vi "Manip_6.vi"() -> ()   [LabVIEW 2020]
uses:
  <vilib>/express/express analysis/Spectral/Block/exnSpectralBlock spectral measurements power poly.vi
  <vilib>/express/express analysis/Spectral/Block/exnSpectralBlock spectral measurements power DDT.vi
  <vilib>/express/express analysis/Spectral/XNode/ExpressSpectralMeasurementsBlockNode.xnode
panel:
  in  "Offset 2":dbl
  in  "Phase 2":dbl
  in  "Offset":dbl
  in  "Phase":dbl
  out "Waveform Graph 2":dynamicdata(graph)
  in  "Freq":dbl(knob) scale=0.0..100.0
  in  "Amp":dbl(knob) scale=0.0..100.0
  in  "Amp":dbl(slide) scale=0.0..100.0
  in  "Freq":dbl(slide) scale=0.0..100.0
  out "Waveform Graph":dynamicdata(graph)
  in  "?":bool
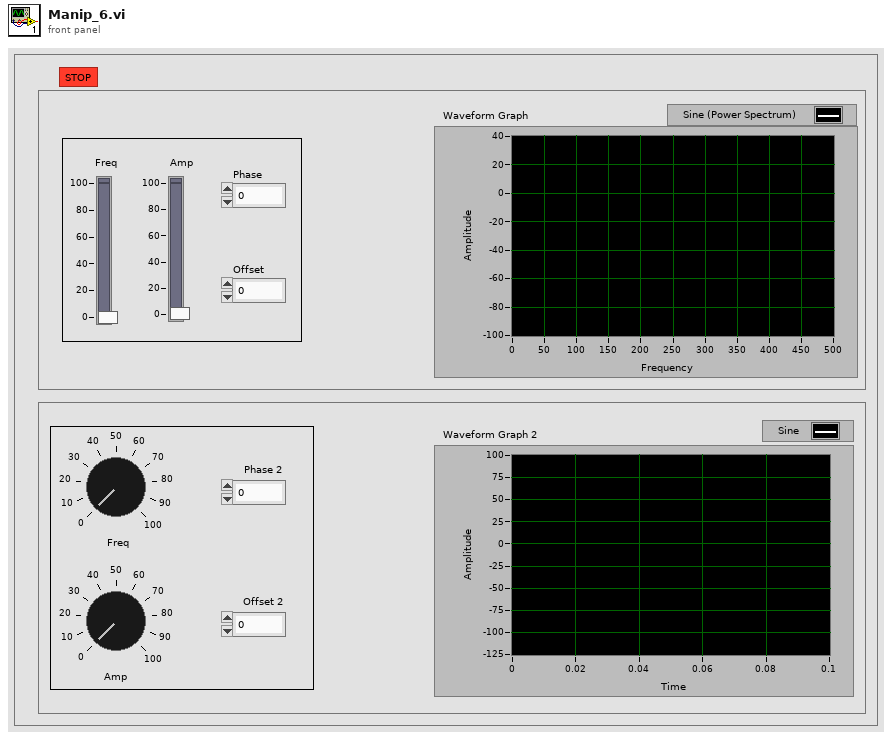
[diagram p1: front panel]
types:
  T1 = cluster{"averaging mode":u16, "weighting mode":u16, "number of averages":u32}
  T2 = cluster{"dB On (F)":bool, "unwrap phase (F)":bool, "convert to degree (F)":bool}
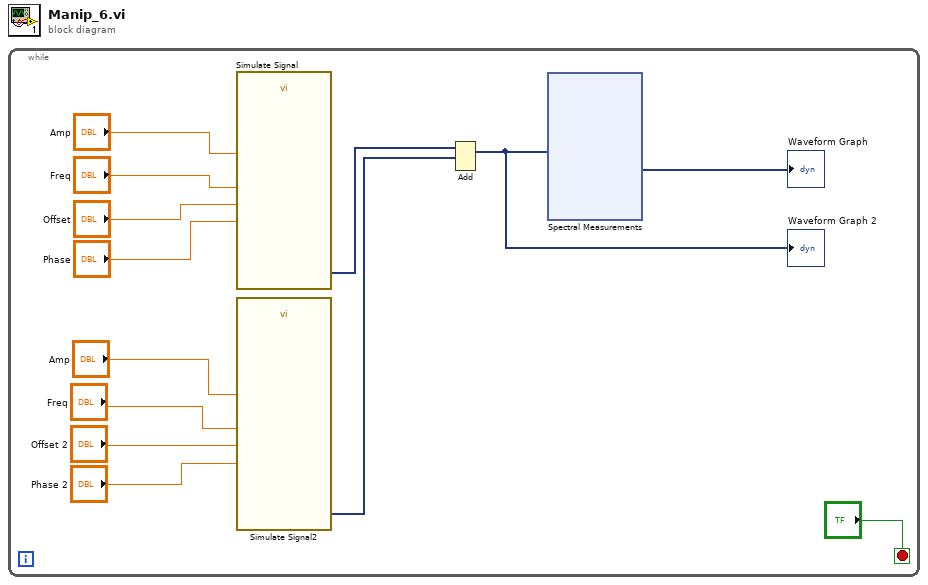
[diagram p0: block diagram]
diagram:
  n1 = while {
    stop <- "?" stop-if-true
    n2 = call "Simulate Signal"("Offset"="Offset", "Frequency"="Freq", "Amplitude"="Amp", "Phase"="Phase") -> ("Sine"=w7:dynamicdata)  [unwired: 10 in, 1 out]
    n3 = call "Simulate Signal2"("Offset"="Offset 2", "Frequency"="Freq", "Amplitude"="Amp", "Phase"="Phase 2") -> ("Sine"=w6:dynamicdata)  [unwired: 10 in, 1 out]
    n4 = Add(1:w6, 2:w7) -> (0:w5:dynamicdata)  [unwired: 1 in, 1 out]
    "Waveform Graph 2" <- w5
    n5 = xnode "Spectral Measurements"("Signals"=w5) -> ("Power Spectrum"=→"Waveform Graph":dynamicdata)  [unwired: 1 in, 1 out]
  }
